vi "Intro_2.vi"() -> ()   [LabVIEW 2018]
panel:
  out "Reponse F":string
  out "Reponse T":string
  in  "b":i8 min=0 max=9
  in  "a":i8 min=0 max=9
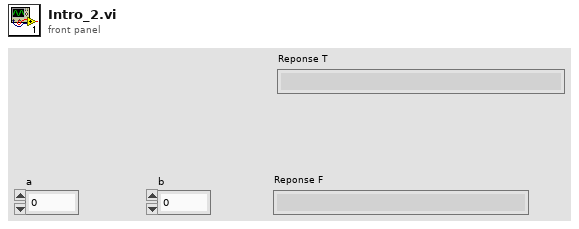
[diagram p1: front panel]
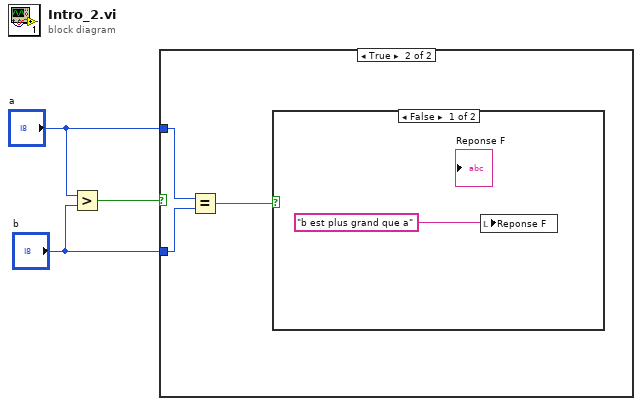
[diagram p0: block diagram]
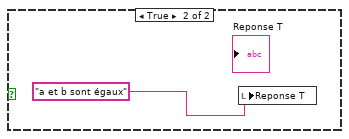
[diagram p3: hidden frame]
diagram:
  n1 = Greater?(x="a", y="b") -> (0:w3:bool)
  n2 = case shown="True" w3 {
    tunnel: "a" -> [_ w5]
    tunnel: "b" -> [_ w6]
    frame False {
    }
    frame True {
      n3 = Equal?(x=w5, y=w6) -> (x = y?=w4:bool)
      n4 = case shown="False" w4 {
        frame False {
          n5 = local write "Reponse F"("b est plus grand que a") -> ()
        }
        frame True {
          n6 = local write "Reponse T"("a et b sont égaux") -> ()
        }
      }
    }
  }
